vi "Proyecto VISA.vi"() -> ()   [LabVIEW 2016]
uses:
  <vilib>/userdefined/High Color/IMAQdx.ctl
  <vilib>/LabVIEW Interface for Arduino/Type Defs/Board Type.ctl
  <vilib>/vision/driver/NI_Vision_Acquisition_Software.lvlib
  <vilib>/vision/NI_Vision_Development_Module.lvlib
  <vilib>/LabVIEW Interface for Arduino/LabVIEW Interface for Arduino.lvlib
panel:
  out "Rampa de X":i32(graph)
  out "Rampa de Y":i32(graph)=45
  out "X":string
  in  "Pos. X":u8=45
  in  "Pos. Y":u8=45
  out "Y":string
  in  "Centro de Y":dbl=228.0
  in  "Centro de X":dbl=282.0
  out "Pos. Servo Y":i32
  out "Pos. Servo X":i32
  out "Objeto Detectado":bool
  out "X":bool
  out "-Y":bool
  out "-X":bool
  out "Y":bool
  out "Valor de Y":sgl
  out "Valor de X":sgl
  in  "Color Plane":i32(ring)=1 items=["Red", "Green", "Blue", "Hue", "Saturation", "Luminance", "Value", "Intensity"]
  in  "stop":bool
  out "Image":T1(plugin-control)
  in  "Settings":T2={"Algorithm"=2, "Number of Matches Requested"=1, "Minimum Match Score"=800.0, "SubPixel Accuracy"=TRUE, "Rotation Angle Ranges"=[], "Show Search Area"=FALSE, "Show Result"=TRUE} {"Rotation Angle Ranges"."End" format="%.1f"; "Rotation Angle Ranges"."Start" format="%.1f"; "Minimum Match Score" min=0 max=1000 format="%.2f"; "Number of Matches Requested" min=1; "Algorithm" items=["All", "Low Discrepancy Sampling", "Grayscale Value Pyramid", "Gradients Pyramid"]}
  in  "Search Rect":T3={"Left"=0, "Top"=0, "Right"=2147483647, "Bottom"=2147483647, "Rotation"=0.0} {"Rotation" format="%.2f"; "Left" scale=0.0..1024.0; "Right" scale=0.0..1024.0}
  in  "File Path":path
  # "Valores en servo X 45°\nSi servo>45°=Abajo\nSi servo<45°=Arriba"
  # "pelotita mide 34"
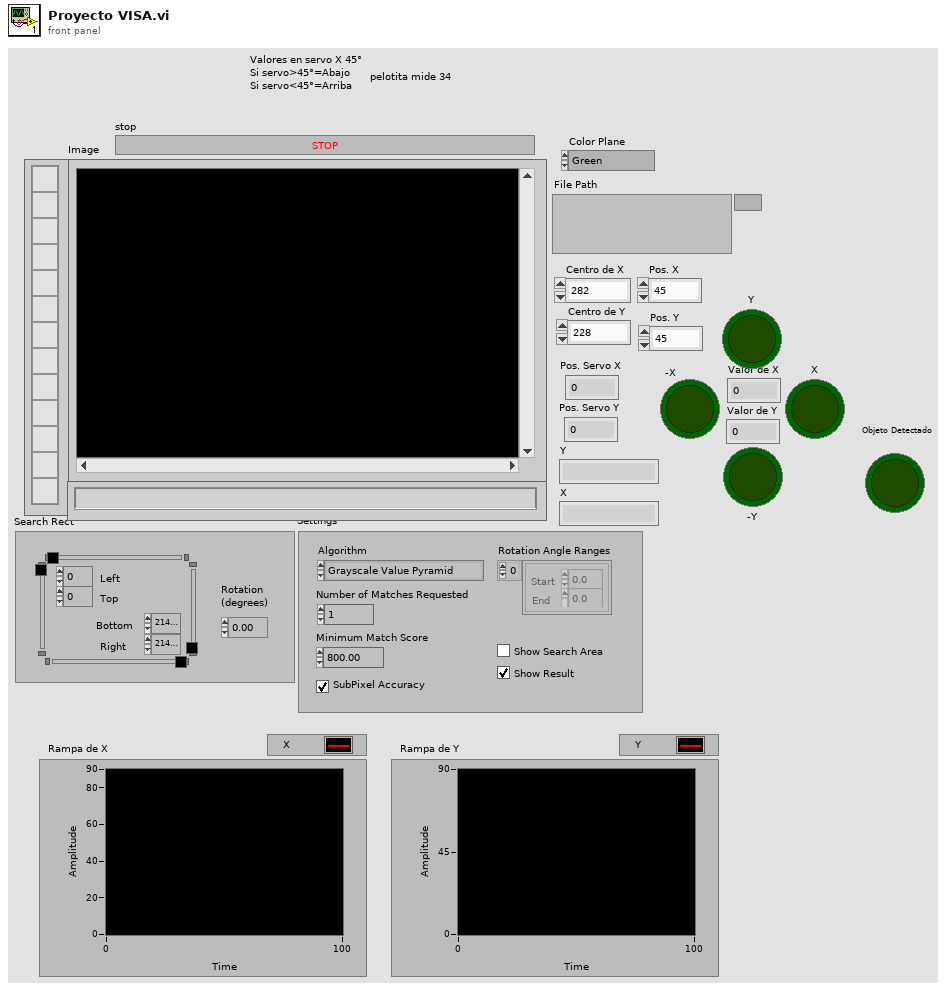
[diagram p1: front panel]
types:
  T1 = typedef "IMAQ Image.ctl" = refnum<image>
  T2 = cluster{"Algorithm":i32, "Number of Matches Requested":i32, "Minimum Match Score":sgl, "SubPixel Accuracy":bool, "Rotation Angle Ranges":cluster{"Start":sgl, "End":sgl}[], "Show Search Area":bool, "Show Result":bool}
  T3 = typedef "IMAQ Rectangle" = cluster{"Left":i32, "Top":i32, "Right":i32, "Bottom":i32, "Rotation":dbl}
  T4 = typedef "LabVIEW Interface for Arduino.lvlib/Board Type.ctl" = enum16{"Uno", "Dimuelanove w/Atmega 328", "Mega 2560"}
  T5 = typedef "IMAQdx.ctl" = refnum<k21>
  T6 = typedef "LabVIEW Interface for Arduino.lvlib/Arduino Resource.ctl" = cluster{"VISA resource":refnum<visa-resource-name>, "Board Type":T4, "Connection Type":enum8{"USB / Serial"}, "Bytes Per Packet (15)":u8}
  T7 = cluster{"Position":cluster{"x":sgl, "y":sgl}, "Angle":sgl, "Scale":sgl, "Score":sgl, "Bounding Box":cluster{"x":sgl, "y":sgl}[]}[]
  T8 = cluster{"Matches (pixel)[0]":cluster{"Position":cluster{"x":sgl, "y":sgl}, "Angle":sgl, "Scale":sgl, "Score":sgl, "Bounding Box":cluster{"x":sgl, "y":sgl}[]}, "Matches (pixel)[1]":cluster{"Position":cluster{"x":sgl, "y":sgl}, "Angle":sgl, "Scale":sgl, "Score":sgl, "Bounding Box":cluster{"x":sgl, "y":sgl}[]}, "Matches (pixel)[2]":cluster{"Position":cluster{"x":sgl, "y":sgl}, "Angle":sgl, "Scale":sgl, "Score":sgl, "Bounding Box":cluster{"x":sgl, "y":sgl}[]}, "Matches (pixel)[3]":cluster{"Position":cluster{"x":sgl, "y":sgl}, "Angle":sgl, "Scale":sgl, "Score":sgl, "Bounding Box":cluster{"x":sgl, "y":sgl}[]}, "Matches (pixel)[4]":cluster{"Position":cluster{"x":sgl, "y":sgl}, "Angle":sgl, "Scale":sgl, "Score":sgl, "Bounding Box":cluster{"x":sgl, "y":sgl}[]}, "Matches (pixel)[5]":cluster{"Position":cluster{"x":sgl, "y":sgl}, "Angle":sgl, "Scale":sgl, "Score":sgl, "Bounding Box":cluster{"x":sgl, "y":sgl}[]}, "Matches (pixel)[6]":cluster{"Position":cluster{"x":sgl, "y":sgl}, "Angle":sgl, "Scale":sgl, "Score":sgl, "Bounding Box":cluster{"x":sgl, "y":sgl}[]}, "Matches (pixel)[7]":cluster{"Position":cluster{"x":sgl, "y":sgl}, "Angle":sgl, "Scale":sgl, "Score":sgl, "Bounding Box":cluster{"x":sgl, "y":sgl}[]}, "Matches (pixel)[8]":cluster{"Position":cluster{"x":sgl, "y":sgl}, "Angle":sgl, "Scale":sgl, "Score":sgl, "Bounding Box":cluster{"x":sgl, "y":sgl}[]}}
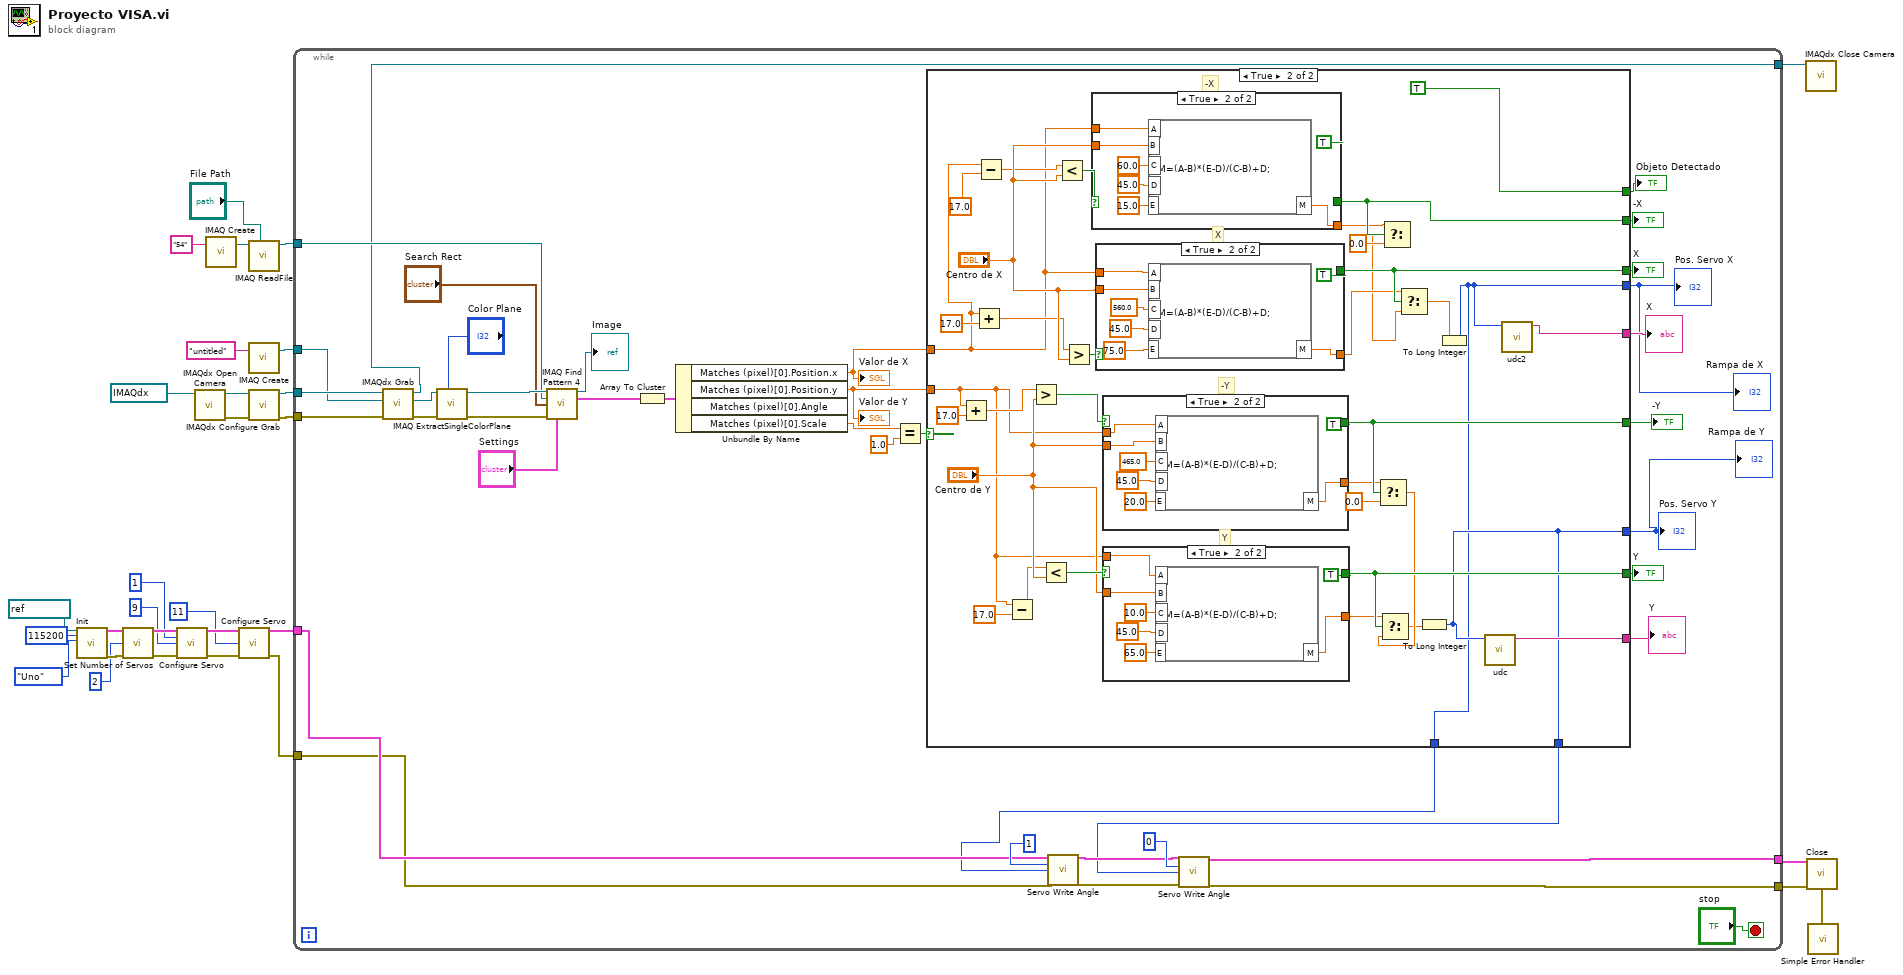
[diagram p0: block diagram]
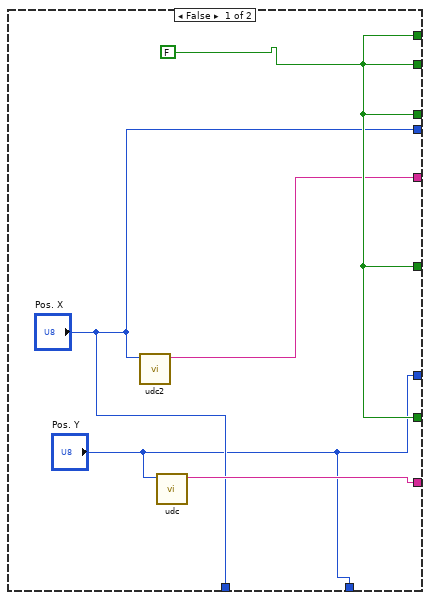
[diagram p2: hidden frame]
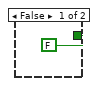
[diagram p3: hidden frame]
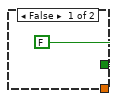
[diagram p4: hidden frame]
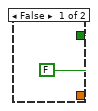
[diagram p5: hidden frame]
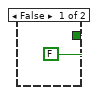
[diagram p6: hidden frame]
diagram:
  n1 = call <vilib>:"Init.vi"("VISA resource"=refnum<visa-resource-name> "COM5", "Baud Rate (115200)"=u32 115200, "Board Type (Uno)"=Board_Type."Uno") -> ("Arduino Resource"=w14:T6, "error out"=w17:errorcluster)  [unwired: 15 in]
  n2 = call <vilib>:"Set Number of Servos.vi"("Arduino Resource"=w14, "Number Of Servos (1)"=u8 2, "error in"=w17) -> ("Arduino Resource"=w13:T6, "error out"=w16:errorcluster)  [unwired: 11 in]
  n3 = call <vilib>:"Configure Servo.vi"("Arduino Resource"=w13, "Servo Number (0)"=u8 1, "DIO Pin (2)"=u8 9, "error in"=w16) -> ("Arduino Resource"=w12:T6, "error out"=w15:errorcluster)  [unwired: 10 in]
  n4 = call <vilib>:"IMAQdx Open Camera.vi"("Session In"=T5 "cam3") -> ("error out"=w30:errorcluster, "Session Out"=w29:T5)  [unwired: 9 in]
  n5 = call "IMAQ Create"("Image Name"="54") -> ("New Image"=w22:T1)  [unwired: 4 in, 1 out]
  n6 = call <vilib>:"Configure Servo.vi"("Arduino Resource"=w12, "DIO Pin (2)"=u8 11, "error in"=w15) -> ("Arduino Resource"=w6:T6, "error out"=w5:errorcluster)  [unwired: 11 in]
  n7 = call "IMAQ ReadFile"("File Path"="File Path", "Image"=w22) -> ("Image Out"=w21:T1)  [unwired: 5 in, 4 out]
  n8 = call "IMAQ Create"("Image Name"="untitled") -> ("New Image"=w24:T1)  [unwired: 4 in, 1 out]
  n9 = call <vilib>:"IMAQdx Configure Grab.vi"("error in"=w30, "Session In"=w29) -> ("error out"=w27:errorcluster, "Session Out"=w28:T5)  [unwired: 8 in]
  n10 = while {
    tunnel: w28 -> [w70]
    tunnel: w27 -> [w69]
    tunnel: w24 -> [w65]
    tunnel: w21 -> [w63]
    tunnel: w5 -> [w35]
    tunnel: w6 -> [w36]
    tunnel: [w44] -> w20
    tunnel: [w34] -> w3
    tunnel: [w33] -> w2
    stop <- "stop" stop-if-true
    n11 = call <vilib>:"IMAQdx Grab.vi"("error in"=w69, "Image In"=w65, "Session In"=w70) -> ("error out"=w68:errorcluster, "Image Out"=w64:T1, "Session Out"=w44:T5)  [unwired: 5 in, 1 out]
    n12 = call "IMAQ ExtractSingleColorPlane"("Color Plane"="Color Plane", "error in (no error)"=w68, "Image Src"=w64) -> ("error out"=w66:errorcluster, "Image Dst Out"=w67:T1)  [unwired: 7 in]
    n13 = call "IMAQ Find Pattern 4"("Image"=w67, "Template"=w63, "Search Rect"="Search Rect", "error in"=w66, "Settings"="Settings") -> ("Image Out"=→"Image":T1, "Matches (pixel)"=w57:T7)  [unwired: 4 in, 5 out]
    n14 = Array To Cluster(array=w57) -> (cluster=w58:T8)
    n15 = Unbundle By Name(w58) -> ("Matches (pixel)[0].Position.x"=w56:sgl, "Matches (pixel)[0].Position.y"=w55:sgl, "Matches (pixel)[0].Scale"=w54:sgl)  [unwired: 1 out]
    "Valor de X" <- w56
    "Valor de Y" <- w55
    n16 = Equal?(x=w54, y=sgl 1.0) -> (x = y?=w52:bool)
    n17 = case shown="True" w52 {
      tunnel: w56 -> [_ w87]
      tunnel: w55 -> [_ w82]
      tunnel: [w75 TRUE] -> w51
      tunnel: [w75 w102] -> w50
      tunnel: [w75 w105] -> w49
      tunnel: [w75 w99] -> w48
      tunnel: [w75 w96] -> w47
      tunnel: [w74 w81] -> w46
      tunnel: [w73 w80] -> w45
      tunnel: ["Pos. Y" w77] -> w43
      tunnel: ["Pos. X" w76] -> w41
      tunnel: ["Pos. Y" w77] -> w32
      tunnel: ["Pos. X" w76] -> w31
      frame False {
        w75 = FALSE
        n18 = call "udc2.vi"("Numeric"="Pos. X") -> ("s? t:f"=w73:string)  [unwired: 10 in]
        n19 = call "udc.vi"("Numeric"="Pos. Y") -> ("s? t:f"=w74:string)  [unwired: 10 in]
      }
      frame True {
        # "X"
        # "-X"
        # "Y"
        # "-Y"
        n20 = Add(x=w82, y=17.0) -> (x+y=w84:dbl)
        n21 = Add(x=w87, y=17.0) -> (x+y=w91:dbl)
        n22 = Subtract(x=w87, y=17.0) -> (x-y=w89:dbl)
        n23 = Subtract(x=w82, y=17.0) -> (x-y=w86:dbl)
        n24 = Greater?(x=w84, y="Centro de Y") -> (0:w109:bool)
        n25 = Less?(x=w86, y="Centro de Y") -> (x < y?=w107:bool)
        n26 = Less?(x=w89, y="Centro de X") -> (x < y?=w108:bool)
        n27 = Greater?(x=w91, y="Centro de X") -> (0:w110:bool)
        n28 = case shown="True" w108 {
          tunnel: [FALSE TRUE] -> w105
          tunnel: "Centro de X" -> [_ w124]
          tunnel: w87 -> [_ w123]
          tunnel: [_ w120] -> w104
          frame False {
          }
          frame True {
            n29 = formula code="M=(A-B)*(E-D)/(C-B)+D;"("A"=w123, "B"=w124, "C"=60.0 ("input variable"), "D"=45.0 ("input variable"), "E"=15.0 ("input variable")) -> ("M"=w120:dbl)
          }
        }
        n30 = case shown="True" w110 {
          tunnel: [FALSE TRUE] -> w102
          tunnel: w87 -> [_ w138]
          tunnel: "Centro de X" -> [_ w137]
          tunnel: [_ w136] -> w101
          frame False {
          }
          frame True {
            n31 = formula code="M=(A-B)*(E-D)/(C-B)+D;"("A"=w138, "B"=w137, "C"=560.0 ("input variable"), "D"=45.0 ("input variable"), "E"=75.0 ("input variable")) -> ("M"=w136:dbl)
          }
        }
        n32 = case shown="True" w109 {
          tunnel: [FALSE TRUE] -> w99
          tunnel: "Centro de Y" -> [_ w132]
          tunnel: [_ w129] -> w98
          tunnel: w82 -> [_ w128]
          frame False {
          }
          frame True {
            n33 = formula code="M=(A-B)*(E-D)/(C-B)+D;"("A"=w128, "B"=w132, "C"=465.0 ("input variable"), "D"=45.0 ("input variable"), "E"=20.0 ("input variable")) -> ("M"=w129:dbl)
          }
        }
        n34 = case shown="True" w107 {
          tunnel: [FALSE TRUE] -> w96
          tunnel: "Centro de Y" -> [_ w116]
          tunnel: w82 -> [_ w115]
          tunnel: [_ w112] -> w95
          frame False {
          }
          frame True {
            n35 = formula code="M=(A-B)*(E-D)/(C-B)+D;"("A"=w115, "B"=w116, "C"=10.0 ("input variable"), "D"=45.0 ("input variable"), "E"=65.0 ("input variable")) -> ("M"=w112:dbl)
          }
        }
        n36 = Select(t=w98, s=w99, f=0.0) -> (s? t:f=w94:dbl)
        n37 = Select(t=w95, s=w96, f=w94) -> (s? t:f=w79:dbl)
        n38 = Select(t=w104, s=w105, f=0.0) -> (s? t:f=w100:dbl)
        n39 = Select(t=w101, s=w102, f=w100) -> (s? t:f=w78:dbl)
        n40 = To Long Integer(number=w79) -> (32bit integer=w77:i32)
        n41 = To Long Integer(number=w78) -> (32bit integer=w76:i32)
        n42 = call "udc.vi"("Numeric"=w77) -> ("s? t:f"=w81:string)  [unwired: 10 in]
        n43 = call "udc2.vi"("Numeric"=w76) -> ("s? t:f"=w80:string)  [unwired: 10 in]
      }
    }
    "Objeto Detectado" <- w51
    "X" <- w50
    "-X" <- w49
    "Y" <- w47
    "-Y" <- w48
    "Y" <- w46
    "X" <- w45
    "Pos. Servo Y" <- w43
    "Pos. Servo X" <- w41
    "Rampa de Y" <- w43
    "Rampa de X" <- w41
    n44 = call <vilib>:"Servo Write Angle.vi"("Arduino Resource"=w36, "Servo Number"=u8 1, "Angle (Degrees)"=w31, "error in"=w35) -> ("Arduino Resource"=w39:T6, "error out"=w38:errorcluster)  [unwired: 10 in]
    n45 = call <vilib>:"Servo Write Angle.vi"("Arduino Resource"=w39, "Servo Number"=u8 0, "Angle (Degrees)"=w32, "error in"=w38) -> ("Arduino Resource"=w34:T6, "error out"=w33:errorcluster)  [unwired: 10 in]
  }
  n46 = call <vilib>:"IMAQdx Close Camera.vi"("Session In"=w20) -> ()  [unwired: 10 in, 1 out]
  n47 = call <vilib>:"Close.vi"("Arduino Resource"=w3, "error in"=w2) -> ("error out"=w4:errorcluster)  [unwired: 13 in]
  n48 = call <vilib>:"Simple Error Handler.vi"("error in (no error)"=w4) -> ()  [unwired: 4 in, 5 out]
